vi "SaveTdms.vi"(0 "object in":refnum<class "MTecSim.lvclass">, 2 "tdms file":refnum<k34>, 3 "group name":string, 5 "error in (no error)":errorcluster) -> (14 "object out":refnum<class "MTecSim.lvclass">, 16 "MtecData":T3={"meTEC_CH2_Temperature Stability"=1, "meTEC_CH2_Act. Output Current [A]"=0.0, "meTEC_CH2_Act. Output Voltage [V]"=0.0, "meTEC_CH2_Object Temperature [°C]"=0.0, "meTEC_CH2_Sink Temperature [°C]"=0.0, "meTEC_CH1_Error Parameter"=0, "meTEC_CH1_Error Instance"=0, "meTEC_CH1_Error No."=0, "meTEC_CH1_Device Status"=1, "meTEC_CH1_Temperature Stability"=1, "meTEC_CH1_Act. Output Current [A]"=0.0, "meTEC_CH1_Act. Output Voltage [V]"=0.0, "meTEC_CH1_Object Temperature [°C]"=0.0, "meTEC_CH1_Sink Temperature [°C]"=0.0} {"meTEC_CH1_Sink Temperature [°C]" format="%.3f"; "meTEC_CH1_Object Temperature [°C]" format="%.3f"; "meTEC_CH1_Act. Output Voltage [V]" format="%.3f"; "meTEC_CH1_Act. Output Current [A]" format="%.3f"; "meTEC_CH1_Temperature Stability" items=["Temperature regulation is not active", "Is not stable", "Is stable"]; "meTEC_CH1_Device Status" items=["Initializing", "Ready", "Run", "Error", "Bootloader", "Reset in Progress"]; "meTEC_CH2_Sink Temperature [°C]" format="%.3f"; "meTEC_CH2_Object Temperature [°C]" format="%.3f"; "meTEC_CH2_Act. Output Voltage [V]" format="%.3f"; "meTEC_CH2_Act. Output Current [A]" format="%.3f"; "meTEC_CH2_Temperature Stability" items=["Temperature regulation is not active", "Is not stable", "Is stable"]}, 19 "error out":errorcluster)   [LabVIEW 2019, in "MTecSim.lvclass"]
uses:
  MTecSim.lvclass
  TEC LabVIEW Control Software v0.14/Source/LV Source/[meerstetter engineering TE Cooling]/TypeDefs/meTEC_ID 1200_Temperature is Stable.ctl
  TEC LabVIEW Control Software v0.14/Source/LV Source/[meerstetter engineering TE Cooling]/TypeDefs/meTEC_ID 104_Device Status.ctl
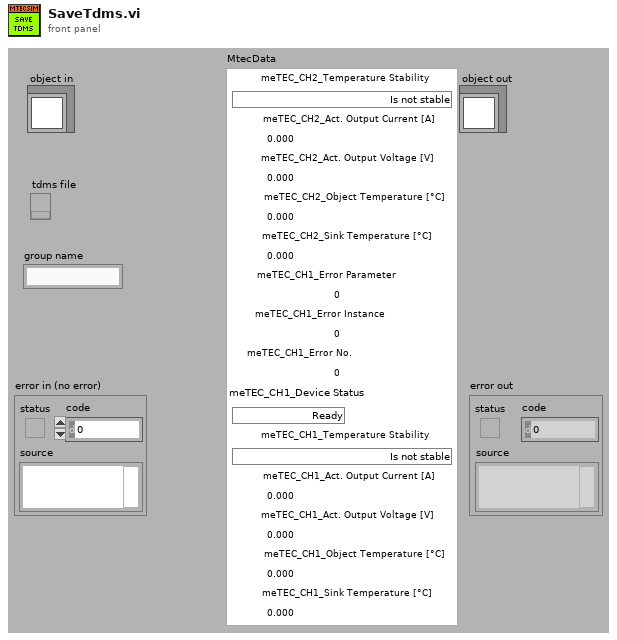
[diagram p1: front panel]
types:
  T1 = typedef "meTEC_ID 1200_Temperature is Stable.ctl" = i32
  T2 = typedef "meTEC_ID 104_Device Status.ctl" = i32
  T3 = cluster{"meTEC_CH2_Temperature Stability":T1, "meTEC_CH2_Act. Output Current [A]":dbl, "meTEC_CH2_Act. Output Voltage [V]":dbl, "meTEC_CH2_Object Temperature [°C]":dbl, "meTEC_CH2_Sink Temperature [°C]":dbl, "meTEC_CH1_Error Parameter":i32, "meTEC_CH1_Error Instance":i32, "meTEC_CH1_Error No.":i32, "meTEC_CH1_Device Status":T2, "meTEC_CH1_Temperature Stability":T1, "meTEC_CH1_Act. Output Current [A]":dbl, "meTEC_CH1_Act. Output Voltage [V]":dbl, "meTEC_CH1_Object Temperature [°C]":dbl, "meTEC_CH1_Sink Temperature [°C]":dbl}
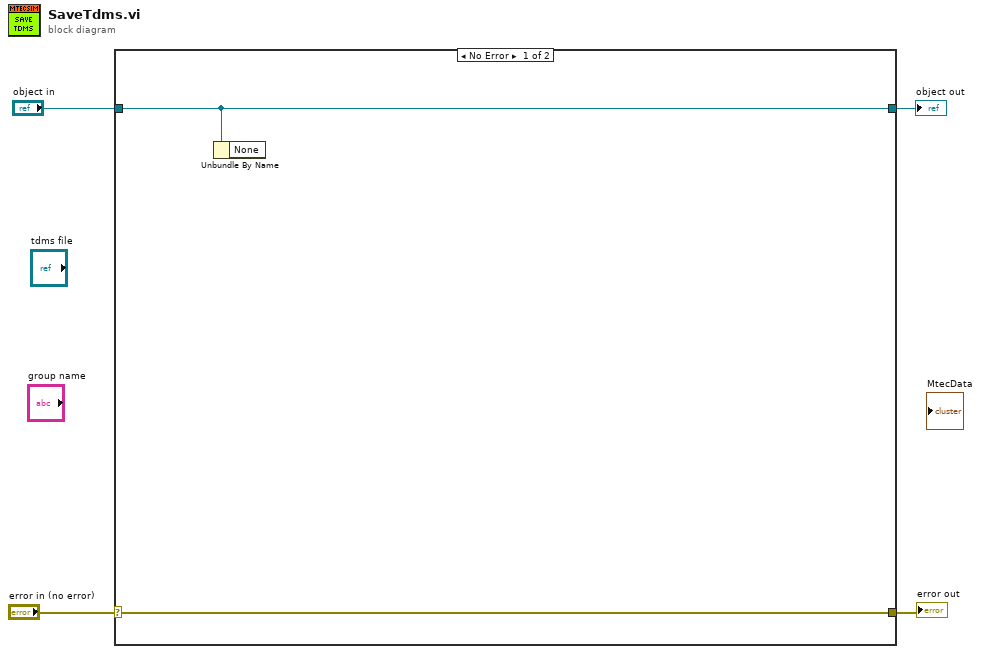
[diagram p0: block diagram]
diagram:
  n1 = case shown="No Error" "error in (no error)" {
    selector: "error in (no error)" -> [w6 w8]
    tunnel: [w6 w8] -> w3
    tunnel: [w5 w7] -> w1
    tunnel: "object in" -> [w5 w7]
    frame No Error {
      n2 = Unbundle By Name(w5) -> ()  [unwired: 1 out]
    }
    frame Error {
    }
  }
  "error out" <- w3
  "object out" <- w1
